vi "Write String.vi"(7 "Output (StdOut)":T1, 8 "error in (no error)":errorcluster, 10 "Text to Write":string, 11 "CLI in":refnum<class "CLI.lvclass">) -> (0 "error out":errorcluster, 3 "CLI out":refnum<class "CLI.lvclass">)   [LabVIEW 2015, in "CLI.lvclass"]
doc: "Writes string data to the command line interface.\n\nNote: This VI does no line handling. You must enter line endings as you want them."
uses:
  CLI.lvclass
  Output.ctl
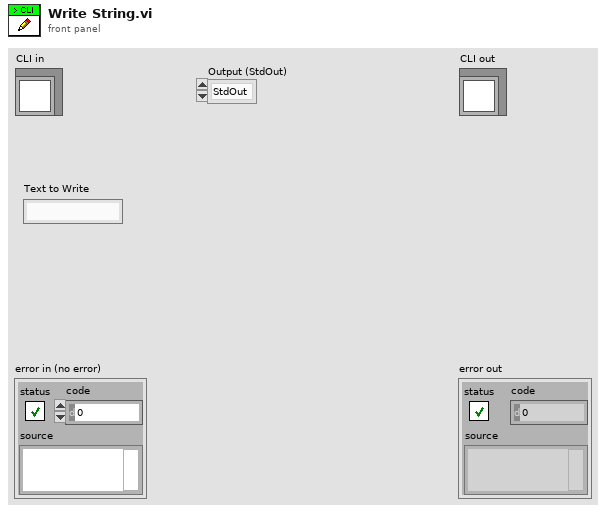
[diagram p1: front panel]
types:
  T1 = typedef "CLI.lvclass/Output.ctl" = enum16{"StdOut", "StdErr"}
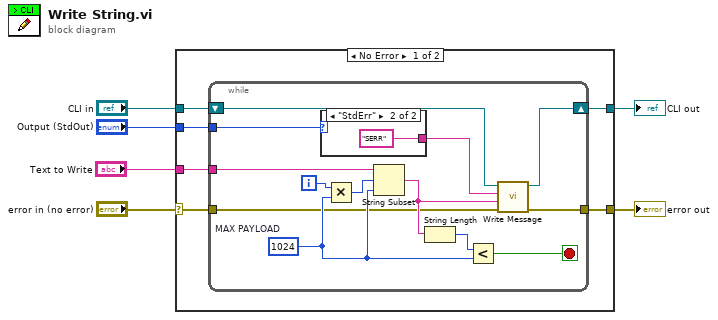
[diagram p0: block diagram]
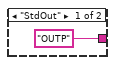
[diagram p2: hidden frame]
diagram:
  n1 = case shown="No Error" "error in (no error)" {
    selector: "error in (no error)" -> [w12 w29]
    tunnel: [w11 w29] -> w5
    tunnel: [w9 w28] -> w3
    tunnel: "CLI in" -> [w10 w28]
    tunnel: "Text to Write" -> [w8 _]
    tunnel: "Output (StdOut)" -> [w7 _]
    frame No Error {
      n2 = while {
        tunnel: w12 -> [w14]
        tunnel: [w25] -> w11
        tunnel: w8 -> [w13]
        shift-right: [w23] -> w9
        shift-left: w10 -> [w24]
        tunnel: w7 -> [w15]
        i -> [w16]
        stop <- w18 stop-if-true
        w20 = 1024  # MAX PAYLOAD
        n3 = case shown="\"StdErr\"" w15 {
          tunnel: ["OUTP" ("Message Type") "SERR" ("Message Type")] -> w22
          frame "StdOut" {
          }
          frame "StdErr" {
          }
        }
        n4 = Multiply(x=w16, y=w20) -> (x*y=w17:i32)
        n5 = String Subset(string=w13, offset (0)=w17, length (rest)=w20) -> (substring=w19:string)
        n6 = String Length(string=w19) -> (length=w21:i32)
        n7 = Less?(x=w21, y=w20) -> (x < y?=w18:bool)
        n8 = call "Write Message.vi"("error in (no error)"=w14, "Message Contents"=w19, "Message Type"=w22, "CLI in"=w24) -> ("error out"=w25:errorcluster, "CLI out"=w23:refnum<class "CLI.lvclass">)  [unwired: 6 in]
      }
    }
    frame Error {
    }
  }
  "error out" <- w5
  "CLI out" <- w3
